vi "example_GArrayUploadFile.vi"() -> ()   [LabVIEW 2020]
uses:
  gclib32.lvlib
  gclibo32.lvlib
panel:
  in  "File Location":string="C:\\Program Files (x86)\\National Instruments\\LabVIEW 2020\\vi.lib\\Galil\\examples\\vi_examples\\example_files\\array_upload.csv"
  in  "Command":string="DM A[5]; A[0]=1; A[1]=2; A[2]=3; A[3]=4; A[4]=5"
  out "Error Out":errorcluster
  in  "IP Address":string="192.168.1.77"
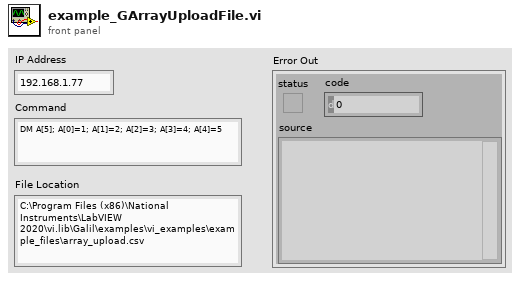
[diagram p1: front panel]
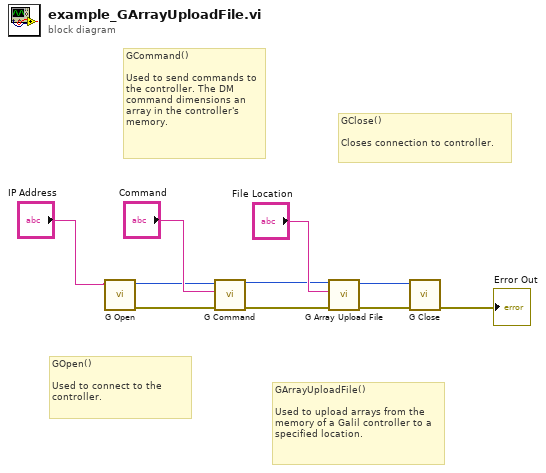
[diagram p0: block diagram]
diagram:
  # "GCommand()\n\nUsed to send commands to the controller. The DM command dimensions an array in the controller's memory."
  # "GClose()\n\nCloses connection to controller."
  # "GArrayUploadFile()\n\nUsed to upload arrays from the memory of a Galil controller to a specified location."
  # "GOpen()\n\nUsed to connect to the controller."
  n1 = call "G Open.vi"("address"="IP Address") -> ("error out"=w1:errorcluster, "g out"=w2:u32)  [unwired: 8 in]
  n2 = call "G Command.vi"("g"=w2, "command"="Command", "error in (no error)"=w1) -> ("g out"=w4:u32, "error out"=w5:errorcluster)  [unwired: 10 in, 1 out]
  n3 = call "G Array Upload File.vi"("error in (no error)"=w5, "file_path"="File Location", "g"=w4) -> ("error out"=w7:errorcluster, "g out"=w8:u32)  [unwired: 7 in]
  n4 = call "G Close.vi"("error in (no error)"=w7, "g"=w8) -> ("error out"=→"Error Out":errorcluster)  [unwired: 9 in]
